vi "Process.vi"(8 "error in (no error)":errorcluster, 10 "Pound in":refnum<class "Pound.lvclass">, 11 "Qbus in":refnum<class "Qbus.lvclass">) -> (0 "error out":errorcluster)   [LabVIEW 2017, in "IrAnalysis.lvlib"]
uses:
  <vilib>/addons/InsightCM/Devices/Shared/Ir/IrAnalysis/IrAnalysis.lvlib
  <vilib>/addons/Qbus/Qbus.lvclass
  <vilib>/NI/Software Watchdog/Pound/Pound.lvclass
  <vilib>/addons/InsightCM/Devices/Shared/Ir/IrAnalysis/controls/config.ctl
  <vilib>/addons/InsightCM/Devices/Shared/Ir/IrAnalysis/controls/roi.ctl
  <vilib>/addons/InsightCM/Devices/Shared/Ir/IrAnalysis/controls/metric.ctl
  <vilib>/addons/InsightCM/MessageBus/Base/controls/MetricDefinitionInstance.ctl
  <vilib>/addons/InsightCM/MessageBus/Base/controls/KeyValuePair.ctl
  <vilib>/addons/TraceLogger/TraceLogger.lvlib
  <vilib>/NI/Software Watchdog/Watchdog/Watchdog.lvclass
  <vilib>/addons/InsightCM/Devices/Shared/Common/DataFlow/DataFlow.lvlib
  <vilib>/addons/InsightCM/Devices/Shared/Common/DataEventCreator/DataEventCreator.lvlib
  <vilib>/addons/InsightCM/Devices/Shared/Ir/IrDataEventCreator/IrDataEventCreator.lvlib
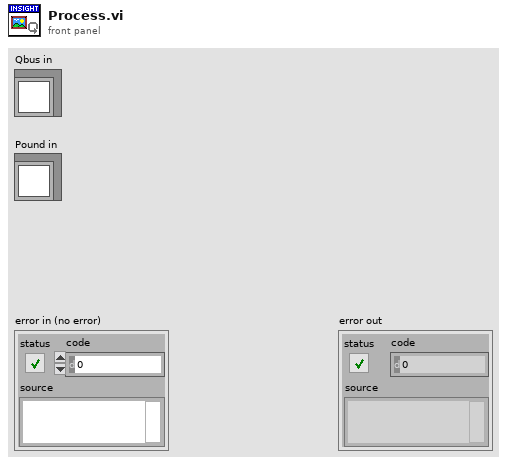
[diagram p1: front panel]
types:
  T1 = typedef "IrAnalysis.lvlib/config.ctl" = cluster{"ROIs":T2[]}
  T2 = typedef "IrAnalysis.lvlib/roi.ctl" = cluster{"name":string, "Id":string, "camera":string, "type":string, "metrics":T3[], "Properties":T5[], "dependency ROI Ids":string[]}
  T3 = typedef "IrAnalysis.lvlib/metric.ctl" = cluster{"Id":string, "Name":string, "instance":T4}
  T4 = typedef "MetricDefinitionInstance.ctl" = cluster{"Id":string, "MetricType":string, "Name":string, "Properties":T5[], "HighRate":bool}
  T5 = typedef "KeyValuePair.ctl" = cluster{"Key":string, "Value":string}
  T6 = typedef "DataEventCreator.lvlib/RegisterTrendPoints.ctl" = cluster{"DataGroup":string, "Trends":T7[]}
  T7 = typedef "DataEventCreator.lvlib/Registry_Trend.ctl" = cluster{"TrendPointId":string, "DataSetName":string, "HighRate":bool, "Always Send":bool}
  T8 = typedef "DataFlow.lvlib/Data.ctl" = cluster{"DataGroup":string, "Waveforms":T9, "Map":T10, "Type":T11}
  T9 = typedef "wfmSGL_DVR.ctl" = refnum<data-value>
  T10 = typedef "PointValueMap.lvlib/PointMap.ctl" = refnum<data-value>
  T11 = typedef "DataFlow.lvlib/Type.ctl" = enum16{"High Rate", "Low Rate", "Burst Mode"}
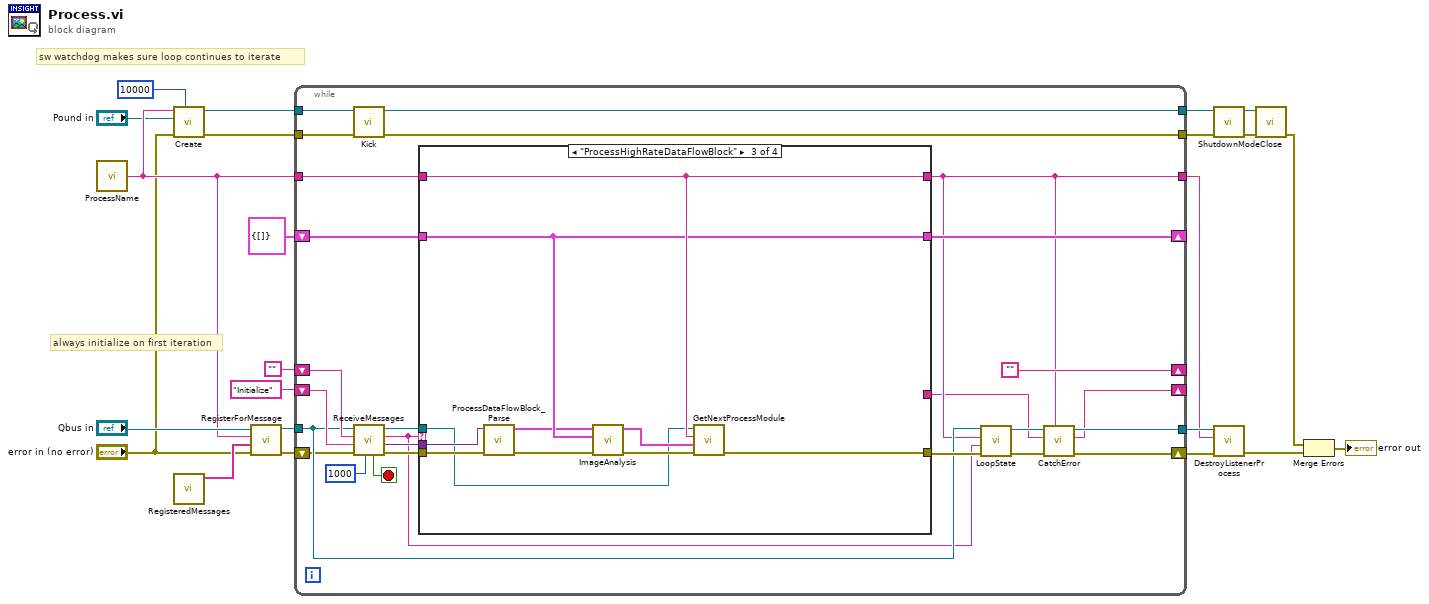
[diagram p0: block diagram]
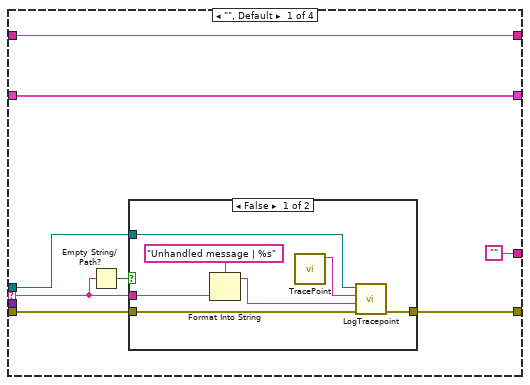
[diagram p2: hidden frame]
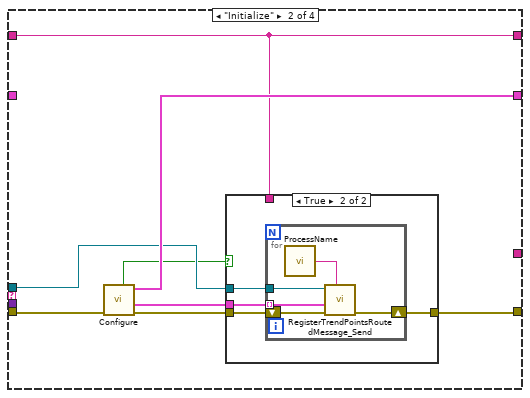
[diagram p4: hidden frame]
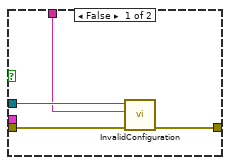
[diagram p5: hidden frame]
diagram:
  # "always initialize on first iteration"
  # "sw watchdog makes sure loop continues to iterate"
  n1 = call <vilib>:"ProcessName.vi"() -> ("process name"=w14:string)  [unwired: 5 in]
  n2 = call <vilib>:"Create.vi"("Execution Timeout (ms)"=u32 10000, "error in (no error)"="error in (no error)", "Pound"="Pound in", "Name"=w14) -> ("error out"=w7:errorcluster, "Watchdog"=w13:refnum<data-value>)  [unwired: 6 in]
  n3 = call <vilib>:"RegisteredMessages.vi"() -> ("registered messages"=w15:string[])  [unwired: 11 in]
  n4 = call <vilib>:"RegisterForMessage.vi"("error in (no error)"="error in (no error)", "message names"=w15, "process name"=w14, "Qbus in"="Qbus in") -> ("error in (no error)"=w22:errorcluster, "Qbus out"=w21:refnum<class "Qbus.lvclass">)  [unwired: 6 in]
  n5 = while {
    shift-right: [""] -> _
    shift-left: "" -> [w48]
    tunnel: w21 -> [w36]
    tunnel: w14 -> [w26]
    tunnel: [w39] -> w19
    tunnel: [w25] -> w18
    shift-right: [w38] -> _
    shift-left: "Initialize" -> [w43]
    shift-right: [w41] -> _
    shift-left: T1 {"ROIs"=[]} ("config") -> [w42]
    tunnel: w13 -> [w35]
    tunnel: [w34] -> w9
    tunnel: w7 -> [w33]
    tunnel: [w31] -> w6
    shift-right: [w40] -> w20
    shift-left: w22 -> [w32]
    stop <- w49 stop-if-true
    n6 = call <vilib>:"Kick.vi"("error in (no error)"=w33, "Watchdog"=w35) -> ("error out"=w31:errorcluster, "Watchdog"=w34:refnum<data-value>)  [unwired: 8 in]
    n7 = call <vilib>:"ReceiveMessages.vi"("Timeout(1000)"=1000 ("milliseconds to wait"), "error in (no error)"=w32, "priority action"=w43, "default action"=w48, "Qbus in"=w36) -> ("error out"=w47:errorcluster, "message value"=w44:variant, "action"=w30:string, "Qbus out"=w45:refnum<class "Qbus.lvclass">, "exit"=w49:bool)  [unwired: 2 in]
    n8 = case shown="\"ProcessHighRateDataFlowBlock\"" w30 {
      selector: w30 -> [w53 _ _ _]
      tunnel: w47 -> [w55 w73 w95 w99]
      tunnel: w45 -> [w51 w68 w87 _]
      tunnel: [w54 w70 w94 w99] -> w37
      tunnel: w44 -> [_ _ w96 _]
      tunnel: w42 -> [w57 _ w90 w98]
      tunnel: [w57 w72 w90 w98] -> w41
      tunnel: [w56 w69 w93 w97] -> w25
      tunnel: w26 -> [w56 w69 w93 w97]
      tunnel: ["" _ _ _] -> w24
      frame "", Default {
        n9 = Empty String/Path?(string/path=w53) -> (empty?=w52:bool)
        n10 = case shown="False" w52 {
          tunnel: [w61 w65] -> w54
          tunnel: w55 -> [w62 w65]
          tunnel: w53 -> [w64 _]
          tunnel: w51 -> [w60 _]
          frame False {
            n11 = Format Into String(format string="Unhandled message | %s", w64) -> (resulting string=w59:string)  [unwired: 2 in, 1 out]
            n12 = call <vilib>:"TracePoint.vi"() -> ("template trace point"=w58:string)  [unwired: 11 in]
            n13 = call <vilib>:"LogTracepoint.vi"("error in (no error)"=w62, "log string"=w59, "tracepoint"=w58, "qbus in"=w60) -> ("error out"=w61:errorcluster)  [unwired: 6 in, 1 out]
          }
          frame True {
          }
        }
      }
      frame "Initialize" {
        n14 = call <vilib>:"Configure.vi"("error in (no error)"=w73) -> ("error out"=w71:errorcluster, "trend point registrations"=w66:T6[], "config"=w72:T1, "valid config"=w67:bool)  [unwired: 7 in]
        n15 = case shown="True" w67 {
          tunnel: w68 -> [w77 w81]
          tunnel: w66 -> [_ w80]
          tunnel: w71 -> [w76 w79]
          tunnel: [w75 w78] -> w70
          tunnel: w69 -> [w74 _]
          frame False {
            n16 = call <vilib>:"InvalidConfiguration.vi"("error in (no error)"=w76, "description"=w74, "Qbus in"=w77) -> ("error out"=w75:errorcluster)  [unwired: 7 in, 1 out]
          }
          frame True {
            n17 = for {
              tunnel: w80 -> [w85] mode=indexing
              shift-right: [w83] -> w78
              shift-left: w79 -> [w84]
              tunnel: w81 -> [w86]
              n18 = call <vilib>:"ProcessName.vi"() -> ("process name"=w82:string)  [unwired: 5 in]
              n19 = call <vilib>:"RegisterTrendPointsRoutedMessage_Send.vi"("data event creator process name"=w82, "error in (no error)"=w84, "register trend"=w85, "Qbus in"=w86) -> ("error out"=w83:errorcluster)  [unwired: 6 in, 1 out]
            }
          }
        }
      }
      frame "ProcessHighRateDataFlowBlock" {
        n20 = call <vilib>:"ProcessDataFlowBlock_Parse.vi"("error in (no error)"=w95, "body"=w96) -> ("error out"=w92:errorcluster, "data"=w89:T8)  [unwired: 8 in]
        n21 = call <vilib>:"ImageAnalysis.vi"("error in (no error)"=w92, "config"=w90, "data"=w89) -> ("error out"=w91:errorcluster, "data out"=w88:T8)  [unwired: 7 in]
        n22 = call <vilib>:"GetNextProcessModule.vi"("error in (no error)"=w91, "data"=w88, "source"=w93, "Qbus in"=w87) -> ("error out"=w94:errorcluster)  [unwired: 6 in, 1 out]
      }
      frame "Exit" {
      }
    }
    n23 = call <vilib>:"LoopState.vi"("error in (no error)"=w37, "loop action"=w30, "process name"=w25, "Qbus in"=w36) -> ("error out"=w28:errorcluster, "Qbus out"=w27:refnum<class "Qbus.lvclass">)  [unwired: 6 in]
    n24 = call <vilib>:"CatchError.vi"("source"=w25, "error in (no error)"=w28, "next action in"=w24, "Qbus in"=w27) -> ("error out"=w40:errorcluster, "next action out"=w38:string, "Qbus out"=w39:refnum<class "Qbus.lvclass">)  [unwired: 5 in]
  }
  n25 = call <vilib>:"ShutdownMode.vi"("error in (no error)"=w6, "Watchdog"=w9) -> ("error out"=w8:errorcluster, "Watchdog"=w10:refnum<data-value>)  [unwired: 8 in]
  n26 = call <vilib>:"DestroyListenerProcess.vi"("error in (no error)"=w20, "process name"=w18, "Qbus in"=w19) -> ("error in (no error)"=w5:errorcluster)  [unwired: 7 in, 1 out]
  n27 = call <vilib>:"Close.vi"("error in (no error)"=w8, "Watchdog"=w10) -> ("error out"=w4:errorcluster)  [unwired: 9 in]
  n28 = Merge Errors(w4, w5) -> (→"error out":errorcluster)
